vi "i q sum.vi"(10 "data in":T1, 11 "data in":T1) -> (3 "output cluster":T1)   [LabVIEW 2021]
doc: "sum 2 IQ datas (I+I =>I ; Q+Q =>Q ; overflow or overflow or +overflow => overflow"
uses:
  <instrlib>/_niInstr/DSP/v1/Shared/Public/IQ Data.ctl
  <vilib>/rvi/FXPMathLib/FxpAdd/XNode/nifxpmath_Add.xnode
  <vilib>/rvi/FXPMathLib/sim/FxpSim.dll
  <instrlib>/_niInstr/DSP/v1/Shared/niInstr DSP v1 Shared.lvlib
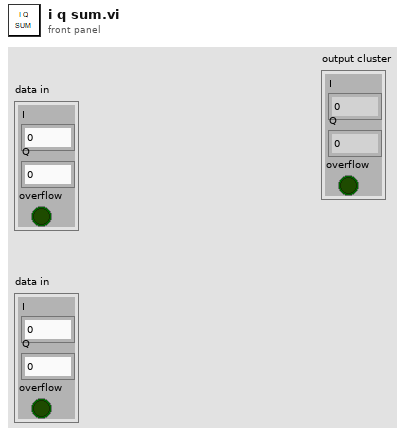
[diagram p1: front panel]
types:
  T1 = typedef "niInstr DSP v1 Shared.lvlib/IQ Data.ctl" = cluster{"I":fxp<+/-,18,1>, "Q":fxp<+/-,18,1>, "overflow":bool}
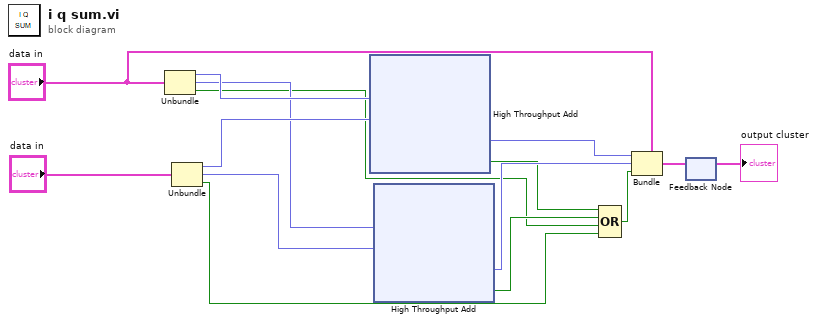
[diagram p0: block diagram]
diagram:
  n1 = Unbundle("data in") -> ("I"=w14:fxp<+/-,18,1>, "Q"=w12:fxp<+/-,18,1>, "overflow"=w6:bool)
  n2 = Unbundle("data in") -> ("I"=w13:fxp<+/-,18,1>, "Q"=w11:fxp<+/-,18,1>, "overflow"=w5:bool)
  n3 = xnode ("High Throughput Add")("x"=w14, "y"=w13) -> ("x+y"=w10:fxp<+/-,18,1>, "operation overflow"=w8:bool)
  n4 = xnode ("High Throughput Add")("x"=w12, "y"=w11) -> ("x+y"=w9:fxp<+/-,18,1>, "operation overflow"=w7:bool)
  n5 = Compound Arithmetic op=OR(w8, w7, w6, w5) -> (w4:bool)
  n6 = Bundle(cluster="data in", "I"=w10, "Q"=w9, "overflow"=w4) -> (w2:T1)
  n7 = feedback-in #1(w2) -> ()
  n8 = feedback #1() -> (→"output cluster":T1)  [unwired: 1 in]
